vi "斐波纳契数列.vi"() -> ()   [LabVIEW 2015]
panel:
  out "斐波那契数组":dbl[](array[numeric])
  in  "数字个数":dbl
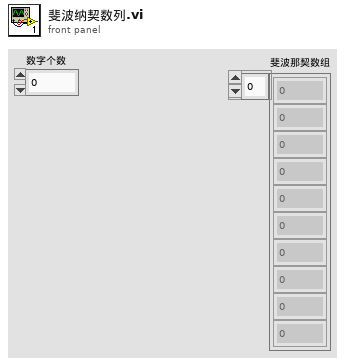
[diagram p1: front panel]
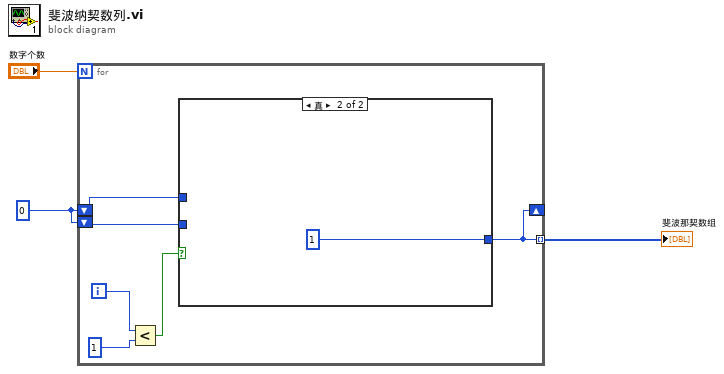
[diagram p0: block diagram]
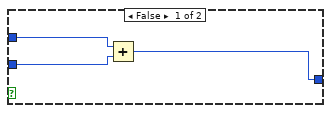
[diagram p2: hidden frame]
diagram:
  w2 = 0
  n1 = for {
    N: "数字个数" -> [_]
    shift-right: [w6] -> _
    shift-left: w2 -> [w8]
    shift-left: w2 -> [w7]
    tunnel: [w6] -> w1 mode=indexing
    i -> [w5]
    n2 = Less?(x=w5, y=1) -> (x < y?=w9:bool)
    n3 = case shown="真" w9 {
      tunnel: [w10 1] -> w6
      tunnel: w8 -> [w12 _]
      tunnel: w7 -> [w11 _]
      frame False {
        n4 = Add(x=w12, y=w11) -> (x+y=w10:i32)
      }
      frame True {
      }
    }
  }
  "斐波那契数组" <- w1
